vi "Display_Trav_Views.vi"(0 "Current Probe Position":dbl[][](array[numeric])=[[15000.0, 0.0, 500.0]] format="%#.1f", 1 "Traverse Name":string, 2 "Currently on point":i32=11, 3 "Open Front Panel":bool, 4 "Error Comments":string, 5 "Crash?":bool, 8 "Row Number":i32=11) -> ()   [LabVIEW 2014]
uses:
  Route_mapping_global.vi
panel:
  out "Warning":string
  in  "Delay in Milliseconds":u32=200 max=10000 step=100
  out "Front View":picture
  out "Side View":picture
  out "Plan View":picture
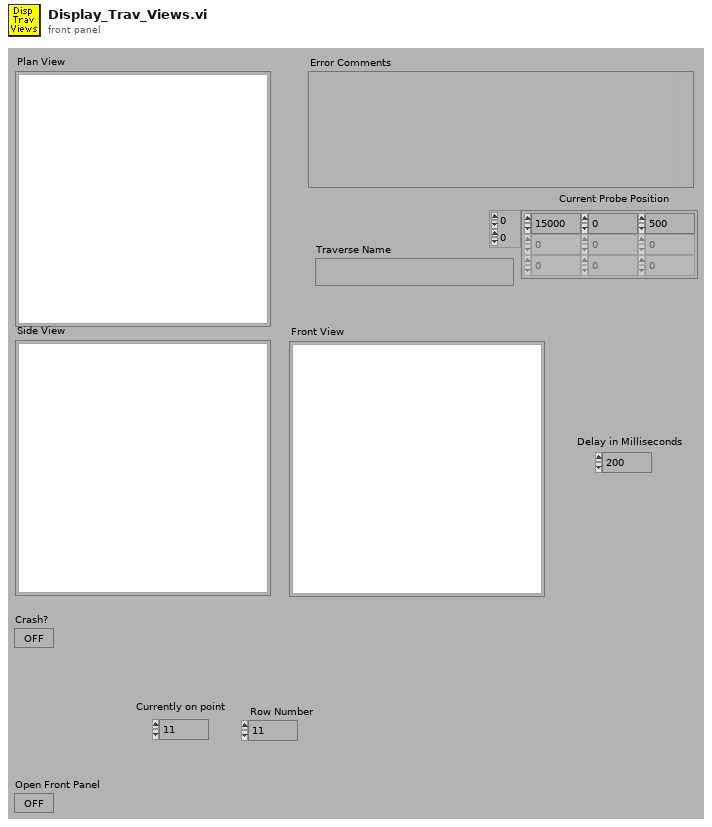
[diagram p1: front panel]
types:
  T1 = typedef "Pict_Plot_Axis.ctl" = cluster{"Width":T2, "Height":T2}
  T2 = typedef "Axis.ctl" = enum16{"X Axis", "X Axis -ve", "Y Axis", "Y Axis -ve", "Z Axis", "Z Axis -ve"}
  T3 = typedef "Box_size.ctl" = cluster{"Max":sgl, "Min":sgl}[]
  T4 = typedef "Exclude_cluster.ctl" = cluster{"Sizes":T3, "Name":string, "Exclude Type":T5}
  T5 = typedef "Exclusion_type.ctl" = enum16{"Exclude completely", "Allow only vertical moves"}
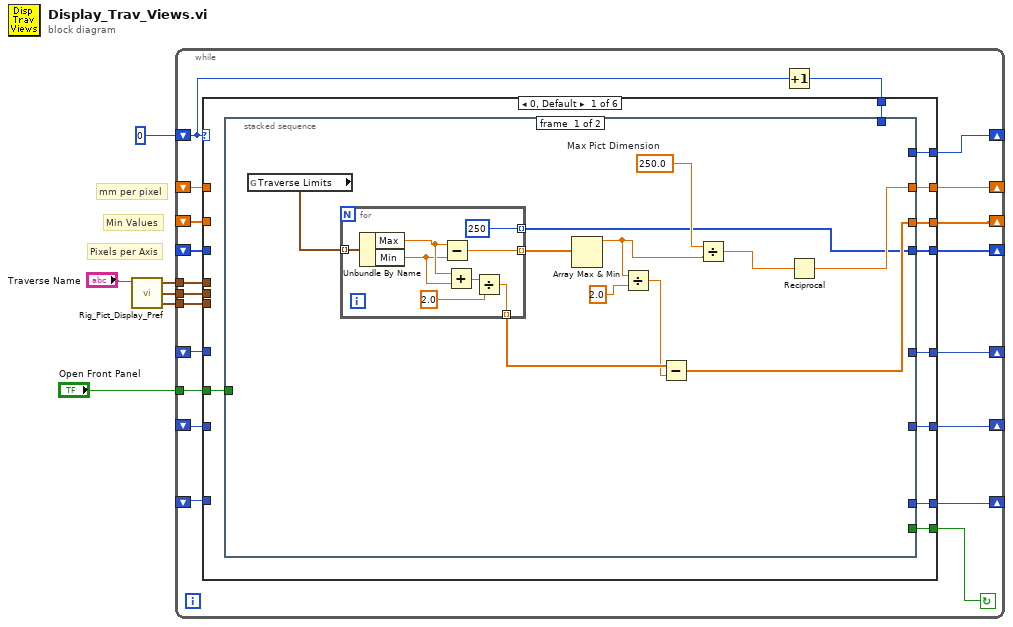
[diagram p0: block diagram]
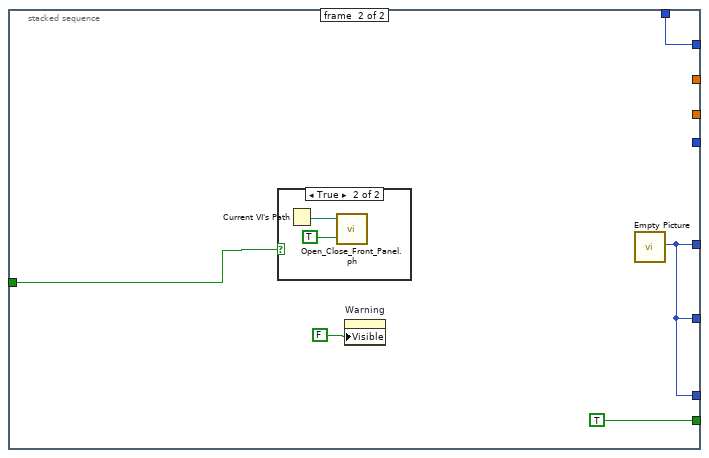
[diagram p2: hidden frame]
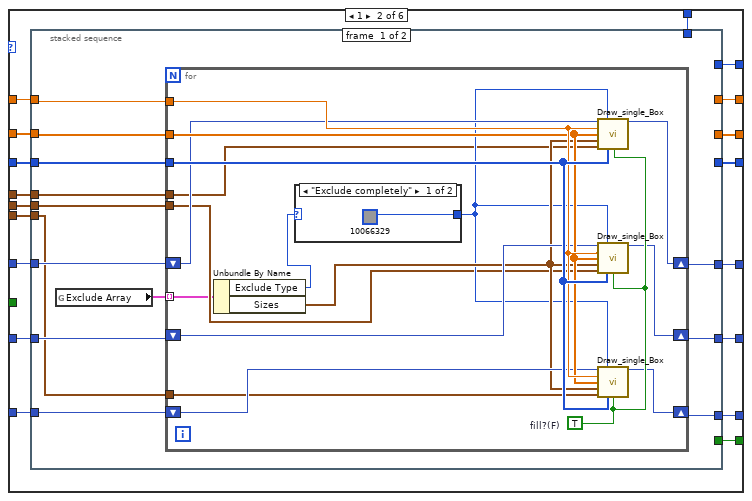
[diagram p4: hidden frame]
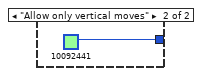
[diagram p5: hidden frame]
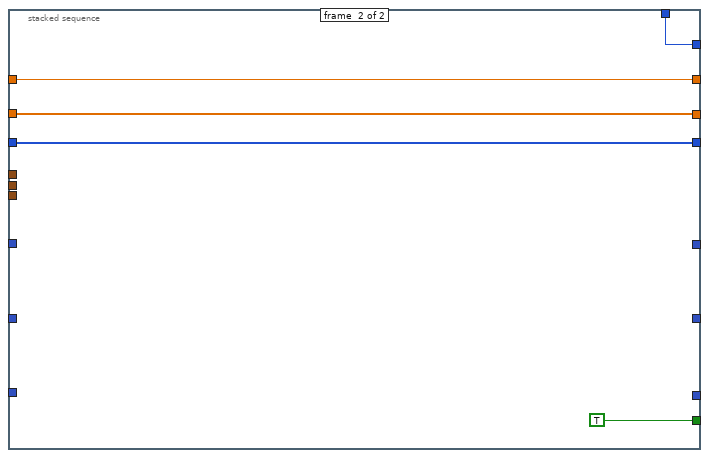
[diagram p6: hidden frame]
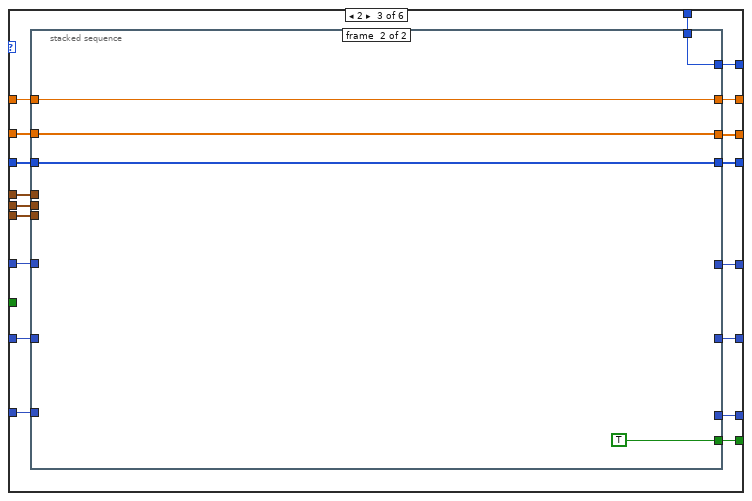
[diagram p7: hidden frame]
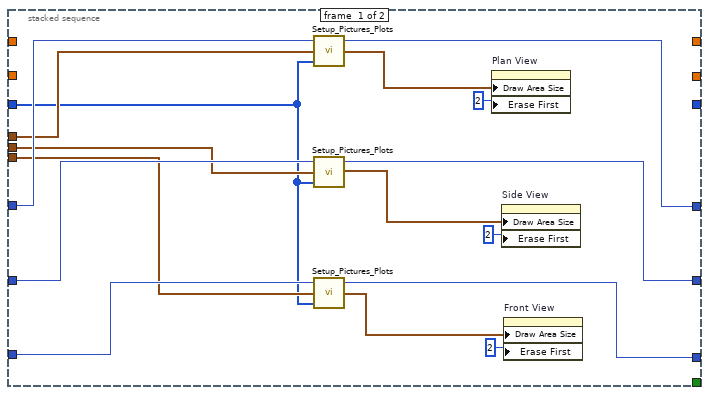
[diagram p8: hidden frame]
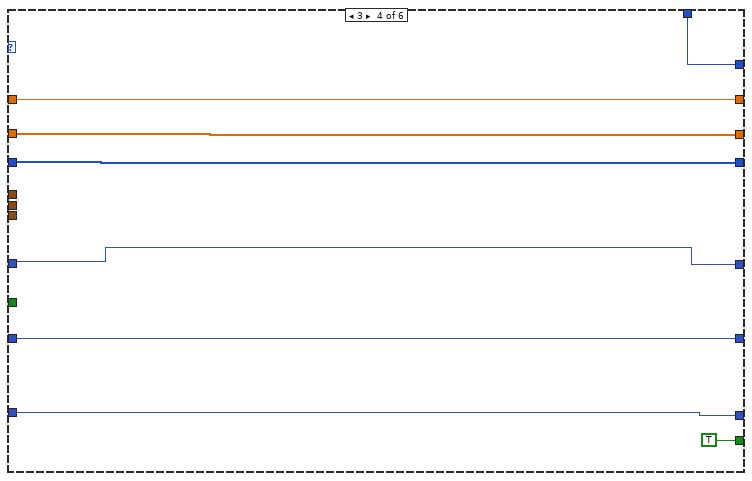
[diagram p9: hidden frame]
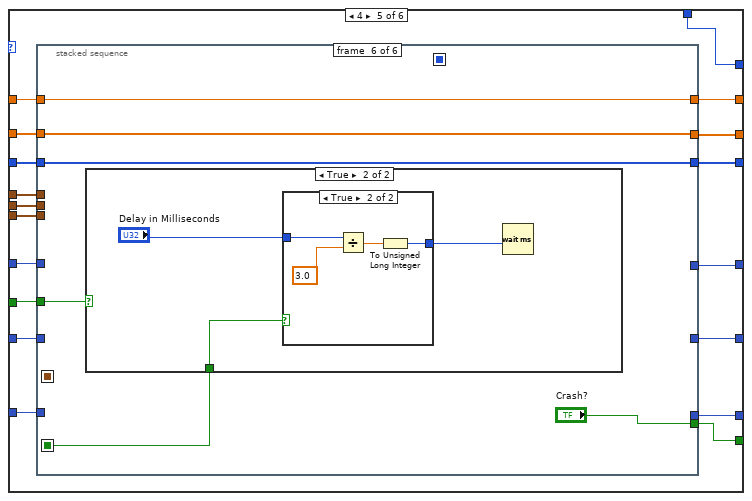
[diagram p10: hidden frame]
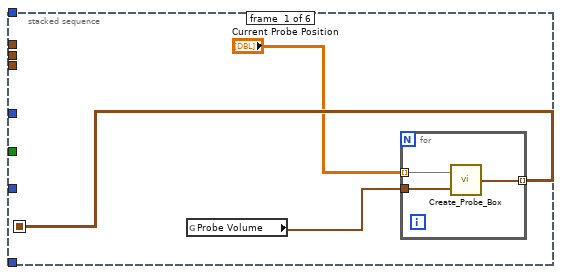
[diagram p11: hidden frame]
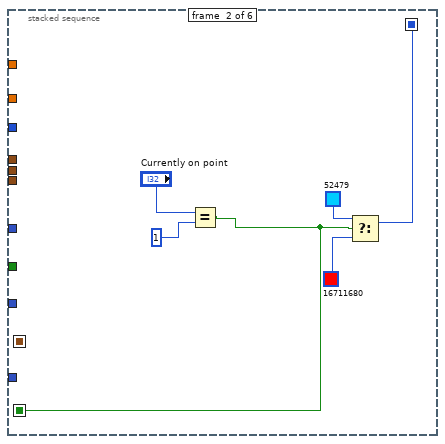
[diagram p12: hidden frame]
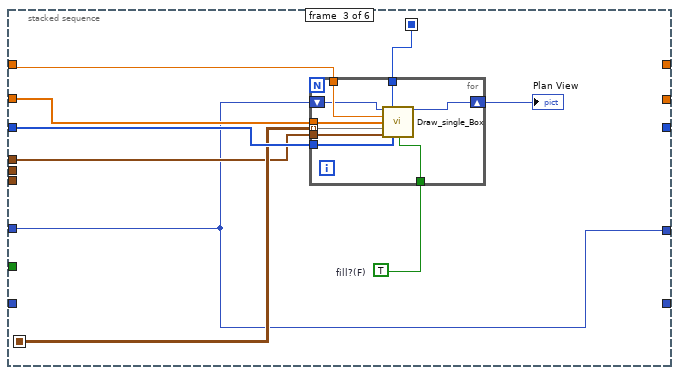
[diagram p13: hidden frame]
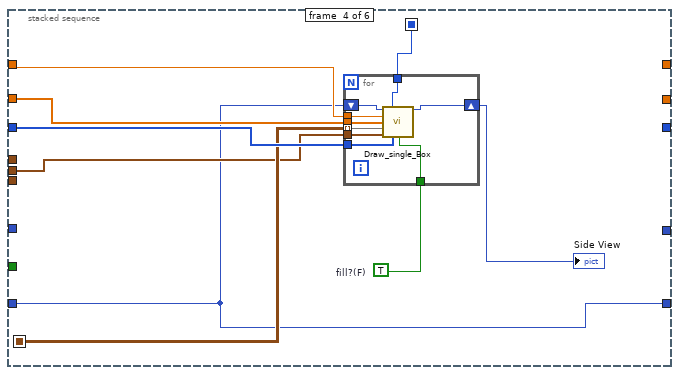
[diagram p14: hidden frame]
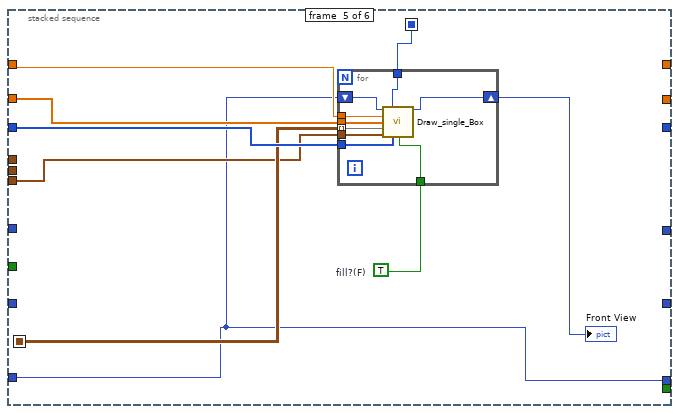
[diagram p15: hidden frame]
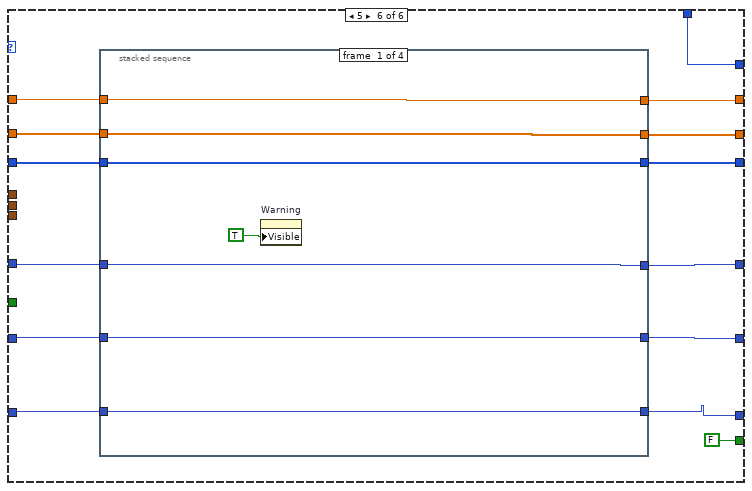
[diagram p18: hidden frame]
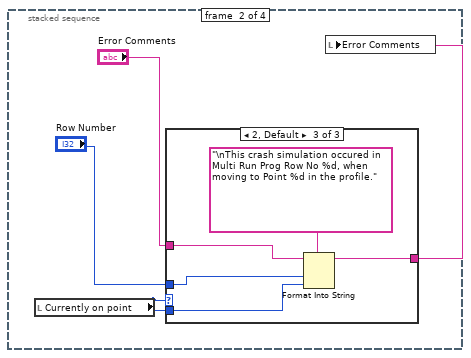
[diagram p19: hidden frame]
diagram:
  # "Min Values"
  # "mm per pixel"
  # "Pixels per Axis"
  n1 = call "Rig_Pict_Display_Pref.vi"("Traverse Name"="Traverse Name") -> ("Plan View"=w5:T1, "Side View"=w4:T1, "Front View"=w3:T1)  [unwired: 5 out]
  n2 = while {
    tunnel: w3 -> [w16]
    tunnel: w4 -> [w17]
    tunnel: w5 -> [w18]
    shift-left: _ -> [w21]
    shift-right: [w10] -> _
    shift-left: _ -> [w20]
    shift-right: [w11] -> _
    shift-left: _ -> [w19]
    shift-right: [w12] -> _
    shift-left: _ -> [w15]
    shift-right: [w25] -> _
    shift-left: _ -> [w14]
    shift-right: [w26] -> _
    shift-left: _ -> [w13]
    shift-right: [w24] -> _
    shift-left: 0 -> [w9]
    shift-right: [w22] -> _
    tunnel: "Open Front Panel" -> [w7]
    stop <- w23 continue-if-true
    n3 = Increment(x=w9) -> (x+1=w8:i32)
    n4 = case shown="0, Default" w9 {
      tunnel: [w36 w80 w135 w162 w182 w273] -> w26
      tunnel: [w35 w79 w134 w161 w181 w271] -> w25
      tunnel: [w34 w78 w133 w163 w180 w275] -> w24
      tunnel: [w33 w66 w132 w158 w169 w269] -> w12
      tunnel: [w32 w65 w131 w160 w168 w267] -> w11
      tunnel: [w31 w64 w130 w159 w167 w265] -> w10
      tunnel: [w30 w77 w129 TRUE ("Crash") w179 FALSE] -> w23
      tunnel: [w29 w76 w128 w164 w166 w263] -> w22
      tunnel: w21 -> [_ w75 w127 w159 w172 w264]
      tunnel: w20 -> [_ w74 w126 w160 w171 w266]
      tunnel: w19 -> [_ w73 w125 w158 w170 w268]
      tunnel: w18 -> [_ w72 w124 _ w178 _]
      tunnel: w17 -> [_ w71 w123 _ w177 _]
      tunnel: w16 -> [_ w70 w122 _ w176 _]
      tunnel: w15 -> [_ w69 w121 w161 w175 w270]
      tunnel: w14 -> [_ w68 w120 w162 w174 w272]
      tunnel: w13 -> [_ w67 w119 w163 w173 w274]
      tunnel: w8 -> [w28 w63 w118 w164 w166 w263]
      tunnel: w7 -> [w27 _ _ _ w165 _]
      frame 0, Default {
        n5 = stacked-sequence {
          tunnel: [w38 _] -> w36
          tunnel: [w37 _] -> w35
          tunnel: [w44 _] -> w34
          tunnel: [_ w58] -> w33
          tunnel: [_ w58] -> w32
          tunnel: [_ w58] -> w31
          tunnel: [_ TRUE] -> w30
          tunnel: [_ w59] -> w29
          tunnel: w28 -> [_ w59]
          tunnel: w27 -> [_ w56]
          frame #0 {
            w45 = 250.0  # Max Pict Dimension
            n6 = global read "Route_mapping_global.vi" "Traverse Limits"() -> (w43:T3)
            n7 = for {
              tunnel: w43 -> [w55] mode=indexing
              tunnel: [w54] -> w46 mode=indexing
              tunnel: [w49] -> w40 mode=indexing
              tunnel: [i16 250 ("16bit integer")] -> w37 mode=indexing
              n8 = Unbundle By Name(w55) -> ("Max"=w53:sgl, "Min"=w52:sgl)
              n9 = Subtract(x=w53, y=w52) -> (x-y=w54:sgl)
              n10 = Add(x=w53, y=w52) -> (x+y=w51:sgl)
              n11 = Divide(x=w51, y=2.0) -> (x/y=w49:dbl)
            }
            n12 = Array Max & Min(array=w46) -> (max value=w41:sgl)  [unwired: 3 out]
            n13 = Divide(x=w41, y=2.0) -> (x/y=w39:dbl)
            n14 = Subtract(x=w40, y=w39) -> (x-y=w38:dbl[])
            n15 = Divide(x=w45, y=w41) -> (x/y=w47:dbl)
            n16 = Reciprocal(x=w47) -> (1/x=w44:dbl)
          }
          frame #1 {
            n17 = case shown="True" w56 {
              frame False {
              }
              frame True {
                n18 = Current VI's Path() -> (path=w62:path)
                n19 = call "Open_Close_Front_Panel.ph.vi"("Front Panel Window:Open"=TRUE, "VI path"=w62) -> ()  [unwired: 2 out]
              }
            }
            n20 = property on="Warning" class="Str"("Visible"=FALSE ("Write Attribute")) -> ()  [unwired: 2 in, 2 out]
            n21 = call "Empty Picture"() -> ("empty picture"=w58:picture)
          }
        }
      }
      frame 1 {
        n22 = stacked-sequence {
          tunnel: [_ w115] -> w80
          tunnel: [_ w116] -> w79
          tunnel: [_ w114] -> w78
          tunnel: [_ TRUE] -> w77
          tunnel: [_ w113] -> w76
          tunnel: w75 -> [w93 _]
          tunnel: w74 -> [w92 _]
          tunnel: w73 -> [w91 _]
          tunnel: w72 -> [w87 _]
          tunnel: w71 -> [w86 _]
          tunnel: w70 -> [w85 _]
          tunnel: w69 -> [w90 w116]
          tunnel: w68 -> [w88 w115]
          tunnel: w67 -> [w89 w114]
          tunnel: [w83 _] -> w66
          tunnel: [w82 _] -> w65
          tunnel: [w81 _] -> w64
          tunnel: w63 -> [_ w113]
          frame #0 {
            n23 = global read "Route_mapping_global.vi" "Exclude Array"() -> (w84:T4[])
            n24 = for {
              shift-right: [w101] -> w83
              shift-left: w91 -> [w106]
              shift-right: [w100] -> w82
              shift-left: w92 -> [w105]
              shift-right: [w99] -> w81
              shift-left: w93 -> [w104]
              tunnel: w90 -> [w109]
              tunnel: w89 -> [w108]
              tunnel: w88 -> [w107]
              tunnel: w87 -> [w97]
              tunnel: w86 -> [w96]
              tunnel: w85 -> [w95]
              tunnel: w84 -> [w94] mode=indexing
              w102 = TRUE  # fill?(F)
              n25 = Unbundle By Name(w94) -> ("Exclude Type"=w110:T5, "Sizes"=w103:T3)
              n26 = case shown="\"Exclude completely\"" w110 {
                tunnel: [u32 10066329 ("color(black)") u32 10092441 ("color(black)")] -> w98
                frame "Exclude completely" {
                }
                frame "Allow only vertical moves" {
                }
              }
              n27 = call "Draw_single_Box.vi"("Picture in"=w106, "color(black)"=w98, "mm Per Pixel"=w108, "Min Values"=w107, "Box Coordinates"=w103, "View"=w97, "Pixels per Axis"=w109, "fill?(F)"=w102) -> ("Picture out"=w101:picture)  [unwired: 7 out]
              n28 = call "Draw_single_Box.vi"("Picture in"=w105, "color(black)"=w98, "mm Per Pixel"=w108, "Min Values"=w107, "Box Coordinates"=w103, "View"=w96, "Pixels per Axis"=w109, "fill?(F)"=w102) -> ("Picture out"=w100:picture)  [unwired: 7 out]
              n29 = call "Draw_single_Box.vi"("Picture in"=w104, "color(black)"=w98, "mm Per Pixel"=w108, "Min Values"=w107, "Box Coordinates"=w103, "View"=w95, "Pixels per Axis"=w109, "fill?(F)"=w102) -> ("Picture out"=w99:picture)  [unwired: 7 out]
            }
          }
          frame #1 {
          }
        }
      }
      frame 2 {
        n30 = stacked-sequence {
          tunnel: [_ w154] -> w135
          tunnel: [_ w155] -> w134
          tunnel: [_ w153] -> w133
          tunnel: [w138 _] -> w132
          tunnel: [w137 _] -> w131
          tunnel: [w136 _] -> w130
          tunnel: [_ TRUE] -> w129
          tunnel: [_ w152] -> w128
          tunnel: w127 -> [w151 _]
          tunnel: w126 -> [w150 _]
          tunnel: w125 -> [w149 _]
          tunnel: w124 -> [w148 _]
          tunnel: w123 -> [w147 _]
          tunnel: w122 -> [w146 _]
          tunnel: w121 -> [w145 w155]
          tunnel: w120 -> [_ w154]
          tunnel: w119 -> [_ w153]
          tunnel: w118 -> [_ w152]
          frame #0 {
            n31 = call "Setup_Pictures_Plots.vi"("Picture Dim"=w145, "Plot Axis"=w148, "Picture In"=w149) -> ("Draw Area Size"=w143:cluster{u32, u32}, "Picture Out"=w138:picture)  [unwired: 1 out]
            n32 = call "Setup_Pictures_Plots.vi"("Picture Dim"=w145, "Plot Axis"=w147, "Picture In"=w150) -> ("Draw Area Size"=w141:cluster{u32, u32}, "Picture Out"=w137:picture)  [unwired: 1 out]
            n33 = call "Setup_Pictures_Plots.vi"("Picture Dim"=w145, "Plot Axis"=w146, "Picture In"=w151) -> ("Draw Area Size"=w139:cluster{u32, u32}, "Picture Out"=w136:picture)  [unwired: 1 out]
            n34 = property on="Plan View" class="Pict"("Draw Area Size"=w143, "Erase First"=u8 2 ("Write Attribute")) -> ()  [unwired: 2 in, 2 out]
            n35 = property on="Side View" class="Pict"("Draw Area Size"=w141, "Erase First"=u8 2 ("Write Attribute")) -> ()  [unwired: 2 in, 2 out]
            n36 = property on="Front View" class="Pict"("Draw Area Size"=w139, "Erase First"=u8 2 ("Write Attribute")) -> ()  [unwired: 2 in, 2 out]
          }
          frame #1 {
          }
        }
      }
      frame 3 {
      }
      frame 4 {
        n37 = stacked-sequence {
          seq-local: [w185 _ _ _ _ _] -> [_ _ w199 w217 w235 _]
          seq-local: [_ w192 _ _ _ _] -> [_ _ w197 w215 w233 _]
          seq-local: [_ w190 _ _ _ _] -> [_ _ _ _ _ w251]
          tunnel: [_ _ _ _ _ w253] -> w182
          tunnel: [_ _ _ _ _ w254] -> w181
          tunnel: [_ _ _ _ _ w252] -> w180
          tunnel: [_ _ _ _ _ "Crash?"] -> w179
          tunnel: w172 -> [_ _ _ _ w232 _]
          tunnel: w171 -> [_ _ _ w214 _ _]
          tunnel: w170 -> [_ _ w196 _ _ _]
          tunnel: w178 -> [_ _ w198 _ _ _]
          tunnel: w177 -> [_ _ _ w216 _ _]
          tunnel: w176 -> [_ _ _ _ w234 _]
          tunnel: w175 -> [_ _ w203 w221 w239 w254]
          tunnel: w174 -> [_ _ w200 w218 w236 w253]
          tunnel: w173 -> [_ _ w202 w220 w238 w252]
          tunnel: [_ _ w196 _ _ _] -> w169
          tunnel: [_ _ _ w214 _ _] -> w168
          tunnel: [_ _ _ _ w232 _] -> w167
          tunnel: w165 -> [_ _ _ _ _ w249]
          frame #0 {
            n38 = global read "Route_mapping_global.vi" "Probe Volume"() -> (w184:T3)
            n39 = for {
              tunnel: [w188] -> w185 mode=indexing
              tunnel: w184 -> [w187]
              tunnel: "Current Probe Position" -> [w186] mode=indexing
              n40 = call "Create_Probe_Box.vi"("Probe Volume"=w187, "Probe Position"=w186) -> ("Current Probe Volume"=w188:T3)
            }
          }
          frame #1 {
            n41 = Equal?(x="Currently on point", y=1) -> (x = y?=w190:bool)
            n42 = Select(t=u32 52479 ("Probe Colour"), s=w190, f=u32 16711680 ("Probe Colour")) -> (s? t:f=w192:u32)
          }
          frame #2 {
            w201 = TRUE  # fill?(F)
            n43 = for {
              tunnel: w203 -> [w212]
              tunnel: w202 -> [w211]
              tunnel: w201 -> [w210]
              tunnel: w200 -> [w209]
              tunnel: w199 -> [w208] mode=indexing
              tunnel: w198 -> [w207]
              tunnel: w197 -> [w206]
              shift-right: [w204] -> w195
              shift-left: w196 -> [w205]
              n44 = call "Draw_single_Box.vi"("Picture in"=w205, "color(black)"=w206, "mm Per Pixel"=w211, "Min Values"=w209, "Box Coordinates"=w208, "View"=w207, "Pixels per Axis"=w212, "fill?(F)"=w210) -> ("Picture out"=w204:picture)  [unwired: 7 out]
            }
            "Plan View" <- w195
          }
          frame #3 {
            w219 = TRUE  # fill?(F)
            n45 = for {
              tunnel: w221 -> [w230]
              tunnel: w220 -> [w229]
              tunnel: w219 -> [w228]
              tunnel: w218 -> [w227]
              tunnel: w217 -> [w226] mode=indexing
              tunnel: w216 -> [w225]
              tunnel: w215 -> [w224]
              shift-right: [w222] -> w213
              shift-left: w214 -> [w223]
              n46 = call "Draw_single_Box.vi"("Picture in"=w223, "color(black)"=w224, "mm Per Pixel"=w229, "Min Values"=w227, "Box Coordinates"=w226, "View"=w225, "Pixels per Axis"=w230, "fill?(F)"=w228) -> ("Picture out"=w222:picture)  [unwired: 7 out]
            }
            "Side View" <- w213
          }
          frame #4 {
            w237 = TRUE  # fill?(F)
            n47 = for {
              tunnel: w239 -> [w248]
              tunnel: w238 -> [w247]
              tunnel: w237 -> [w246]
              tunnel: w236 -> [w245]
              tunnel: w235 -> [w244] mode=indexing
              tunnel: w234 -> [w243]
              tunnel: w233 -> [w242]
              shift-right: [w240] -> w231
              shift-left: w232 -> [w241]
              n48 = call "Draw_single_Box.vi"("Picture in"=w241, "color(black)"=w242, "mm Per Pixel"=w247, "Min Values"=w245, "Box Coordinates"=w244, "View"=w243, "Pixels per Axis"=w248, "fill?(F)"=w246) -> ("Picture out"=w240:picture)  [unwired: 7 out]
            }
            "Front View" <- w231
          }
          frame #5 {
            n49 = case shown="True" w249 {
              tunnel: w251 -> [_ w257]
              frame False {
              }
              frame True {
                n50 = case shown="True" w257 {
                  tunnel: "Delay in Milliseconds" -> [w258 w262]
                  tunnel: [w258 w259] -> w255
                  frame False {
                  }
                  frame True {
                    n51 = Divide(x=w262, y=3.0) -> (x/y=w260:dbl)
                    n52 = To Unsigned Long Integer(number=w260) -> (unsigned 32bit integer=w259:u32)
                  }
                }
                n53 = Wait (ms)(milliseconds to wait=w255) -> ()  [unwired: 1 out]
              }
            }
          }
        }
      }
      frame 5 {
        n54 = stacked-sequence {
          tunnel: [w283 _ _ _] -> w275
          tunnel: w274 -> [w283 _ _ _]
          tunnel: [w282 _ _ _] -> w273
          tunnel: w272 -> [w282 _ _ _]
          tunnel: [w281 _ _ _] -> w271
          tunnel: w270 -> [w281 _ _ _]
          tunnel: [w280 _ _ _] -> w269
          tunnel: w268 -> [w280 _ _ _]
          tunnel: [w279 _ _ _] -> w267
          tunnel: w266 -> [w279 _ _ _]
          tunnel: [w278 _ _ _] -> w265
          tunnel: w264 -> [w278 _ _ _]
          frame #0 {
            n55 = property on="Warning" class="Str"("Visible"=TRUE ("Write Attribute")) -> ()  [unwired: 2 in, 2 out]
          }
          frame #1 {
            n56 = local read "Currently on point"() -> (w285:i32)
            n57 = case shown="2, Default" w285 {
              tunnel: "Row Number" -> [_ w293 w295]
              tunnel: "Error Comments" -> [w288 w290 w297]
              tunnel: [w288 w289 w296] -> w286
              tunnel: w285 -> [_ _ w294]
              frame -1 {
              }
              frame 1 {
                n58 = Decrement(x=w293) -> (x-1=w292:i32)
                n59 = Format Into String(format string="\nThis crash simulation occured when moving the traverse from the last position in Row %d to the first position in Row %d." ("Format String"), initial string=w290, w292, w293) -> (resulting string=w289:string)  [unwired: 1 in, 1 out]
              }
              frame 2, Default {
                n60 = Format Into String(format string="\nThis crash simulation occured in Multi Run Prog Row No %d, when moving to Point %d in the profile." ("Format String"), initial string=w297, w295, w294) -> (resulting string=w296:string)  [unwired: 1 in, 1 out]
              }
            }
            n61 = local write "Error Comments"(w286) -> ()
          }
          frame #2 {
            n62 = for {
              N: 5 -> [_]
              shift-right: [w305] -> _
              shift-left: TRUE -> [w306]
              n63 = Select(t="Crash", s=w306, f="! ! ! ! ! ") -> (s? t:f=→"Warning":string)
              n64 = Wait (ms)(milliseconds to wait=u32 500) -> ()  [unwired: 1 out]
              n65 = Not(x=w306) -> (.not. x?=w305:bool)
            }
          }
          frame #3 {
            n66 = Stop(stop? (T)=TRUE) -> ()
          }
        }
      }
    }
  }
